vi "Number Widget.vi"(8 "Error In":errorcluster, 11 "Post-Bundled Subclass":refnum<class "Number Widget.lvclass">) -> (0 "Error Out":errorcluster, 3 "New Number Widget":refnum<class "Number Widget.lvclass">)   [LabVIEW 2014, in "5. Creating a User-Defined Signal.lvlib" / "Number Widget.lvclass"]
doc: "Constructs a new Number Widget.\n\n\nCopyright (c) 2019 Sze Howe Koh.\nThis code is licensed under the MIT license."
uses:
  Number Widget.lvclass
  <vilib>/addons/LQ/Qt Widgets/QBoxLayout/Direction.ctl
  <vilib>/addons/LQ/Qt Widgets/QFrame/Shadow.ctl
  <vilib>/addons/LQ/Qt Widgets/QFrame/Shape.ctl
  Number Widget.lvclass/Number Widget.ctl
  <vilib>/addons/LQ/Qt Widgets/QFrame/setFrameShadow.vi
  <vilib>/addons/LQ/Qt Widgets/QFrame/setFrameShape.vi
  <vilib>/addons/LQ/LQ Core/LQCoreEngine/_Polymorphic Instances/Connect_SignatureIn_Signal.vi
  <vilib>/addons/LQ/LQ Core/LQCoreEngine/_Polymorphic Instances/Connect_SignatureIn_QtSlot.vi
  <vilib>/addons/LQ/Qt Widgets/QLCDNumber/QLCDNumber.lvclass
  <vilib>/addons/LQ/Qwt/QwtSlider/QwtSlider.lvclass
  <vilib>/addons/LQ/Qt Widgets/QBoxLayout/QBoxLayout.lvclass
  <vilib>/addons/LQ/Qt Widgets/QWidget/QWidget.lvclass
  <vilib>/addons/LQ/LQ Core/LQObject/LQObject.lvclass
  <vilib>/addons/LQ/LQ Core/LQCoreEngine/LQCoreEngine.lvclass
  <vilib>/addons/LQ/Qt Widgets/QFrame/QFrame.lvclass
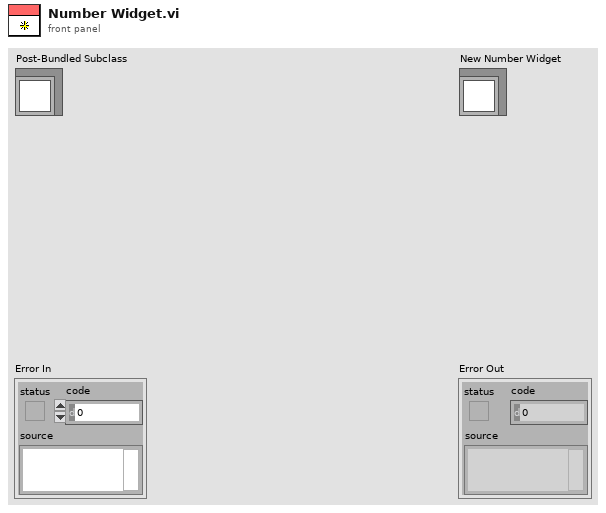
[diagram p1: front panel]
types:
  T1 = typedef "QFrame.lvclass/Shape.ctl" = i32
  T2 = typedef "QFrame.lvclass/Shadow.ctl" = i32
  T3 = typedef "QBoxLayout.lvclass/Direction.ctl" = i32
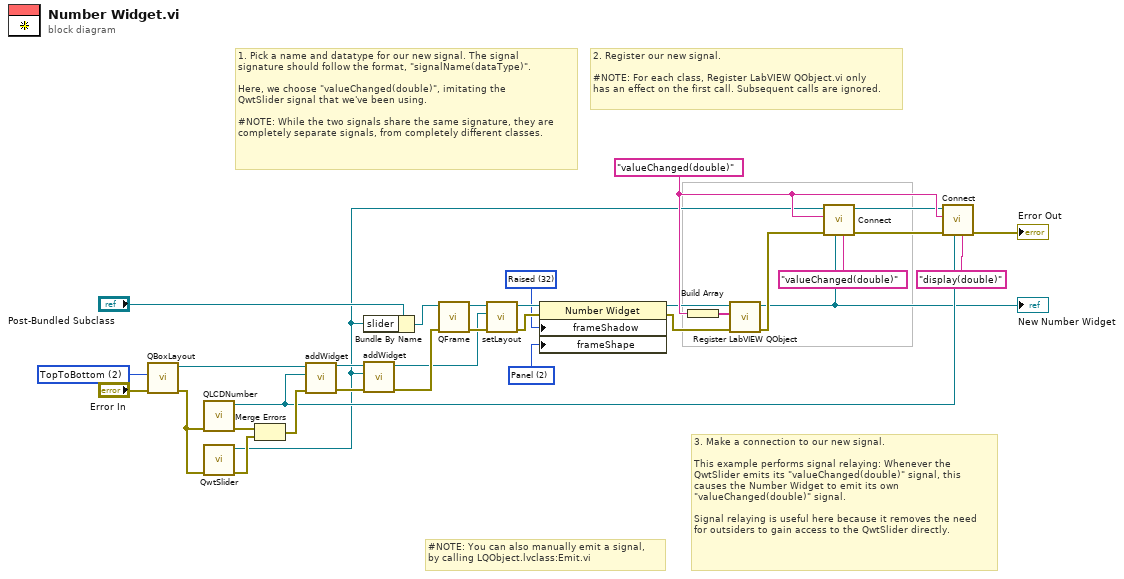
[diagram p0: block diagram]
diagram:
  w1 = T1 2 items=["NoFrame", "Box", "Panel", "HLine", "VLine", "StyledPanel"] ("frameShape")
  w2 = T2 32 items=["Plain"=16, "Raised"=32, "Sunken"=48] ("frameShadow")
  w10 = T3 2 items=["LeftToRight", "RightToLeft", "TopToBottom", "BottomToTop"] ("direction")
  w15 = "valueChanged(double)" ("Signal")
  # "#NOTE: You can also manually emit a signal,\nby calling LQObject.lvclass:Emit.vi"
  # "1. Pick a name and datatype for our new signal. The signal \nsignature should follow the format, \"signalName(dataType)\".\n\nHere, we choose \"valueChanged(double)\", imitating the\nQwtSlider signal that we've been using.\n\n#NOTE: While the two signals share the same signature, they are\ncompletely separate signals, from completely different classes."
  # "3. Make a connection to our new signal.\n\nThis example performs signal relaying: Whenever the\nQwtSlider emits its \"valueChanged(double)\" signal, this\ncauses the Number Widget to emit its own\n\"valueChanged(double)\" signal.\n\nSignal relaying is useful here because it removes the need\nfor outsiders to gain access to the QwtSlider directly."
  # "2. Register our new signal. \n\n#NOTE: For each class, Register LabVIEW QObject.vi only\nhas an effect on the first call. Subsequent calls are ignored."
  n1 = call <vilib>:"QBoxLayout.vi"("Error In"="Error In", "direction"=w10) -> ("Error Out"=w20:errorcluster, "New QBoxLayout"=w29:refnum<class "QBoxLayout.lvclass">)  [unwired: 8 in]
  n2 = call <vilib>:"QLCDNumber.vi"("Error In"=w20) -> ("Error Out"=w18:errorcluster, "New QLCDNumber"=w17:refnum<class "QLCDNumber.lvclass">)  [unwired: 9 in]
  n3 = call <vilib>:"QwtSlider.vi"("Error In"=w20) -> ("Error Out"=w19:errorcluster, "New QwtSlider"=w14:refnum<class "QwtSlider.lvclass">)  [unwired: 9 in]
  n4 = Merge Errors(w18, w19) -> (w30:errorcluster)
  n5 = call <vilib>:"addWidget.vi"("Error In"=w30, "widget"=w17, "QBoxLayout In"=w29) -> ("Error Out"=w25:errorcluster, "QBoxLayout Out"=w28:refnum<class "QBoxLayout.lvclass">)  [unwired: 7 in]
  n6 = Bundle By Name(cluster="Post-Bundled Subclass", "slider"=w14) -> (w9:refnum<class "Number Widget.lvclass">)
  n7 = call <vilib>:"addWidget.vi"("Error In"=w25, "widget"=w14, "QBoxLayout In"=w28) -> ("Error Out"=w32:errorcluster, "QBoxLayout Out"=w26:refnum<class "QBoxLayout.lvclass">)  [unwired: 7 in]
  n8 = call <vilib>:"QFrame.vi"("Error In"=w32, "Post-Bundled Subclass"=w9) -> ("Error Out"=w31:errorcluster, "New QFrame"=w27:refnum<class "Number Widget.lvclass">)  [unwired: 8 in]
  n9 = call <vilib>:"setLayout.vi"("Error In"=w31, "layout"=w26, "QWidget In"=w27) -> ("Error Out"=w4:errorcluster, "QWidget Out"=w6:refnum<class "Number Widget.lvclass">)  [unwired: 7 in]
  n10 = property class="Number Widget"(reference=w6, error in=w4, "frameShadow"=w2, "frameShape"=w1) -> (reference out=w5:refnum<class "Number Widget.lvclass">, error out=w3:errorcluster)
  n11 = Build Array(w15) -> (w21:string[])
  n12 = call <vilib>:"Register LabVIEW QObject.vi"("Error In"=w3, "New Signals"=w21, "Custom LQObject In"=w5) -> ("Error Out"=w8:errorcluster, "Custom LQObject Out"=w7:refnum<class "Number Widget.lvclass">)  [unwired: 7 in]
  "New Number Widget" <- w7
  n13 = call-poly <vilib>:"Connect.vi"("Relay Signal Signature"="valueChanged(double)" ("Signal"), "Relay Object"=w7, "Error In"=w8, "Source Signal Signature"=w15, "Sender In"=w14) -> ("Error Out"=w12:errorcluster, "Sender Out"=w13:refnum<class "QwtSlider.lvclass">)  [unwired: 5 in]
  n14 = call-poly <vilib>:"Connect.vi"("Slot Signature"="display(double)" ("Slot"), "Receiver"=w17, "Error In"=w12, "Signal Signature"=w15, "Sender In"=w13) -> ("Error Out"=→"Error Out":errorcluster)  [unwired: 5 in, 1 out]
